vi "QuitLabVIEW.vi"   [LabVIEW 2015]
doc: "Quits LabVIEW after a certain delay."
uses:
  Argument Parser/Option Class/Option Configuration.ctl
  Argument Parser/Option Class/Argument Type.ctl
  CLI Class/CLI.lvclass
  Argument Parser/Option Set Class/Option Set.lvclass
  Argument Parser/Option Class/Option.lvclass
types:
  T1 = typedef "Option Parser.lvlib/Option.lvclass/Option Configuration.ctl" = cluster{"Option Type":T2, "Option Labels":string[], "Key":string, "Description":string, "Required":bool, "Default Value":string}
  T2 = typedef "Option Parser.lvlib/Option.lvclass/Argument Type.ctl" = enum16{"flag", "value"}
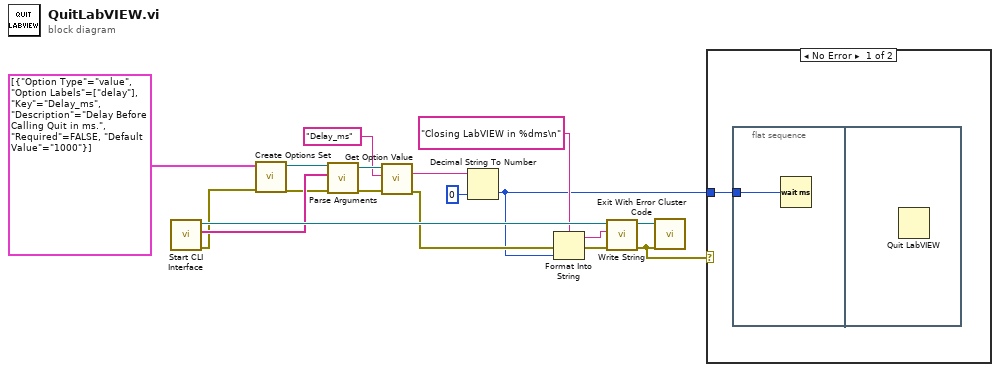
[diagram p0: block diagram]
diagram:
  n1 = call "Start CLI Interface.vi"() -> ("error out"=w11:errorcluster, "Custom Parameters"=w16:string[], "CLI out"=w17:refnum<class "CLI.lvclass">)  [unwired: 8 in, 1 out]
  n2 = call "Create Options Set.vi"("error in (no error)"=w11, "Options"=T1[] [{"Option Type"=enum."value", "Option Labels"=["delay"], "Key"="Delay_ms", "Description"="Delay Before Calling Quit in ms.", "Required"=FALSE, "Default Value"="1000"}]) -> ("error out"=w12:errorcluster, "Option Set out"=w13:refnum<class "Option Set.lvclass">)  [unwired: 8 in]
  n3 = call "Parse Arguments.vi"("error in (no error)"=w12, "Arguments"=w16, "Option Set in"=w13) -> ("error out"=w15:errorcluster, "Option Set out"=w14:refnum<class "Option Set.lvclass">)  [unwired: 5 in, 2 out]
  n4 = call "Get Option Value.vi"("error in (no error)"=w15, "Option Key"="Delay_ms", "Option Set in"=w14) -> ("error out"=w9:errorcluster, "Value"=w7:string)  [unwired: 5 in, 2 out]
  n5 = Decimal String To Number(string=w7, default (0L)=u32 0 ("default (0 I32)")) -> (number=w3:u32)  [unwired: 1 in, 1 out]
  n6 = Format Into String(format string="Closing LabVIEW in %dms\n", error in=w9, w3) -> (resulting string=w4:string, error out=w6:errorcluster)  [unwired: 1 in]
  n7 = call "Write String.vi"("error in (no error)"=w6, "Text to Write"=w4, "CLI in"=w17) -> ("error out"=w1:errorcluster, "CLI out"=w18:refnum<class "CLI.lvclass">)  [unwired: 7 in]
  n8 = call "Exit With Error Cluster Code.vi"("error in (no error)"=w1, "CLI in"=w18) -> ()  [unwired: 9 in, 1 out]
  n9 = case shown="No Error" w1 {
    tunnel: w3 -> [w19 _]
    frame No Error {
      n10 = flat-sequence {
        tunnel: w19 -> [w20]
        frame #0 {
          n11 = Wait (ms)(milliseconds to wait=w20) -> ()  [unwired: 1 out]
        }
        frame #1 {
          n12 = Quit LabVIEW() -> ()  [unwired: 1 in]
        }
      }
    }
    frame Error {
      # "Don't exit if there is an error.\n\nIt's probably been run directly by accident."
    }
  }
